vi "integrate_resonance_simple.vi"(5 "waiting iterations per pixel":u32, 7 "integration iterations per pixel":u32, 9 "iteration counter in":u32, 10 "sampling values in":T2, 11 "integration cluster in":T1) -> (1 "finished?":bool, 2 "iteration counter out":u32, 3 "integration cluster out":T1)   [LabVIEW 2010]
uses:
  common_typedefs/channels_cluster.ctl
  integration_cluster.ctl
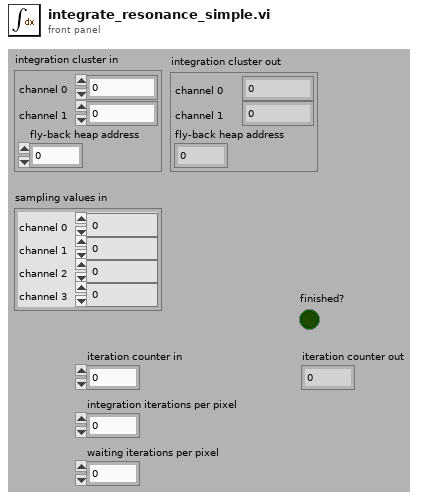
[diagram p1: front panel]
types:
  T1 = typedef "integration_cluster.ctl" = cluster{"channel 0":u32, "channel 1":u32, "fly-back heap address":u32}
  T2 = typedef "channels_cluster.ctl" = cluster{"channel 0":u32, "channel 1":u32, "channel 2":u32, "channel 3":u32}
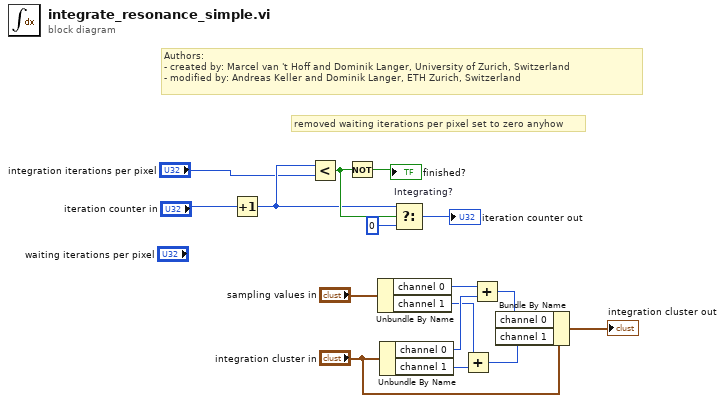
[diagram p0: block diagram]
diagram:
  # "removed waiting iterations per pixel set to zero anyhow"
  # "Authors: \n- created by: Marcel van 't Hoff and Dominik Langer, University of Zurich, Switzerland\n- modified by: Andreas Keller and Dominik Langer, ETH Zurich, Switzerland"
  n1 = Increment(x="iteration counter in") -> (x+1=w12:u32)
  n2 = Less?(x=w12, y="integration iterations per pixel") -> (x < y?=w13:bool)
  n3 = Not(x=w13) -> (.not. x?=→"finished?":bool)
  n4 = Unbundle By Name("sampling values in") -> ("channel 0"=w7:u32, "channel 1"=w5:u32)
  n5 = Unbundle By Name("integration cluster in") -> ("channel 0"=w6:u32, "channel 1"=w4:u32)
  n6 = Select "Integrating?"(t=w12, s=w13, f=u32 0) -> (s? t:f=→"iteration counter out":u32)
  n7 = Add(x=w5, y=w4) -> (x+y=w2:u32)
  n8 = Add(x=w7, y=w6) -> (x+y=w3:u32)
  n9 = Bundle By Name(cluster="integration cluster in", "channel 0"=w3, "channel 1"=w2) -> (→"integration cluster out":T1)
